vi "RestoreUISettings.vi"(8 "Error In":errorcluster, 11 "UI References":T1) -> (0 "Error Out":errorcluster)   [LabVIEW 2017, in "Client.lvlib" / "UI_API.lvlib"]
uses:
  UI_API.lvlib
  NI_LVConfig.lvlib
  Client.lvlib
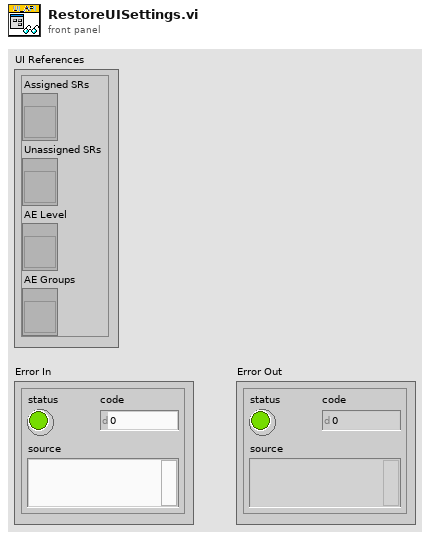
[diagram p1: front panel]
types:
  T1 = cluster{"Assigned SRs":refnum<vi>, "Unassigned SRs":refnum<vi>, "AE Level":refnum<vi>, "AE Groups":refnum<vi>}
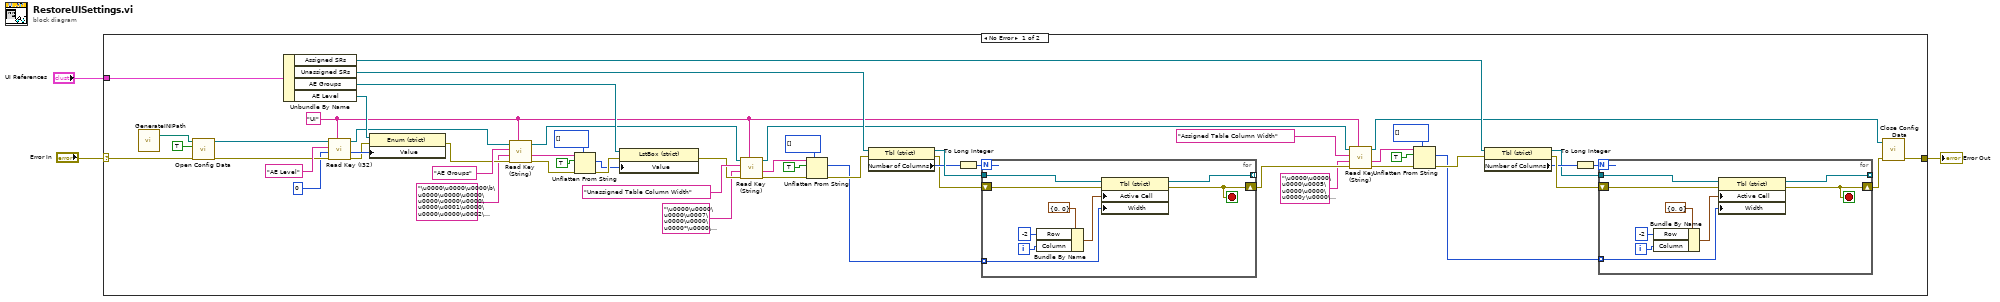
[diagram p0: block diagram]
diagram:
  n1 = case shown="No Error" "Error In" {
    selector: "Error In" -> [w58 w78]
    tunnel: "UI References" -> [w57 _]
    tunnel: [w54 w78] -> w1
    frame No Error {
      w24 = "UI" ("section")
      n2 = call "GenerateINIPath.vi"() -> ("INI Path"=w4:path)  [unwired: 11 in]
      n3 = call "Open Config Data.vi"("error in (no error)"=w58, "create file if necessary (T)"=TRUE ("create file if necessary? (T)"), "configuration file path"=w4) -> ("error out"=w45:errorcluster, "refnum"=w48:refnum<k1>)  [unwired: 6 in, 1 out]
      n4 = Unbundle By Name(w57) -> ("Assigned SRs"=w12:refnum<vi>, "Unassigned SRs"=w53:refnum<vi>, "AE Groups"=w55:refnum<vi>, "AE Level"=w56:refnum<vi>)
      n5 = call "Read Key (I32).vi"("section"=w24, "error in (no error)"=w45, "default value"=0, "key"="AE Level", "refnum"=w48) -> ("error out"=w44:errorcluster, "value"=w46:i32, "refnum out"=w40:refnum<k1>)  [unwired: 3 in, 1 out]
      n6 = property class="Enum (strict)"(reference=w56, error in=w44, "Value"=w46) -> (error out=w41:errorcluster)  [unwired: 1 out]
      n7 = call "Read Key (String).vi"("section"=w24, "error in (no error)"=w41, "default value"="\u0000\u0000\u0000\b\u0000\u0000\u0000\u0000\u0000\u0000\u0000\u0001\u0000\u0000\u0000\u0002\u0000\u0000\u0000\u0003\u0000\u0000\u0000\u0004\u0000\u0000\u0000\u0005\u0000\u0000\u0000\u0006\u0000\u0000\u0000\u0007", "key"="AE Groups", "refnum"=w40) -> ("error out"=w37:errorcluster, "value"=w38:string, "refnum out"=w32:refnum<k1>)  [unwired: 3 in, 1 out]
      n8 = Unflatten From String(type=i32[] [] ("Value"), binary string=w38, data includes array or string size? (T)=TRUE, error in (no error)=w37) -> (value=w35:i32[], error out=w36:errorcluster)  [unwired: 1 in, 1 out]
      n9 = property class="LstBox (strict)"(reference=w55, error in=w36, "Value"=w35) -> (error out=w33:errorcluster)  [unwired: 1 out]
      n10 = call "Read Key (String).vi"("section"=w24, "error in (no error)"=w33, "default value"="\u0000\u0000\u0000\u0007\u0000\u0000\u0000*\u0000\u0000\u0000F\u0000\u0000\u0000L\u0000\u0000\u0001\u0000\u0000\u0001\u0013\u0000\u0000\u0000E\u0000\u0000\u0000Z", "key"="Unassigned Table Column Width", "refnum"=w32) -> ("error out"=w28:errorcluster, "value"=w29:string, "refnum out"=w22:refnum<k1>)  [unwired: 3 in, 1 out]
      n11 = Unflatten From String(type=u32[] [], binary string=w29, data includes array or string size? (T)=TRUE, error in (no error)=w28) -> (value=w26:u32[], error out=w27:errorcluster)  [unwired: 1 in, 1 out]
      n12 = property class="Tbl (strict)"(reference=w53, error in=w27) -> (reference out=w52:refnum<vi>, error out=w49:errorcluster, "Number of Columns"=w51:u32)
      n13 = To Long Integer(number=w51) -> (32bit integer=w50:i32)
      n14 = for {
        N: w50 -> [_]
        shift-right: [w71] -> w25
        shift-left: w49 -> [w72]
        tunnel: w52 -> [w77]
        tunnel: [w73] -> _ mode=indexing
        tunnel: w26 -> [w70] mode=indexing
        i -> [w69]
        stop <- w71 stop-if-true
        n15 = Bundle By Name(cluster=cluster{"Row":i32, "Column":i32} {"Row"=0, "Column"=0} ("Active Cell:Active Cell"), "Row"=-2, "Column"=w69) -> (w74:cluster{"Row":i32, "Column":i32})
        n16 = property class="Tbl (strict)"(reference=w77, error in=w72, "Active Cell"=w74, "Width"=w70) -> (reference out=w73:refnum<vi>, error out=w71:errorcluster)
      }
      n17 = call "Read Key (String).vi"("section"=w24, "error in (no error)"=w25, "default value"="\u0000\u0000\u0000\u0005\u0000\u0000\u0000y\u0000\u0000\u0000;\u0000\u0000\u0001n\u0000\u0000\u0001\u0000\u0000\u0001\u0013", "key"="Assigned Table Column Width", "refnum"=w22) -> ("error out"=w15:errorcluster, "value"=w14:string, "refnum out"=w9:refnum<k1>)  [unwired: 3 in, 1 out]
      n18 = Unflatten From String(type=u32[] [], binary string=w14, data includes array or string size? (T)=TRUE, error in (no error)=w15) -> (value=w11:u32[], error out=w13:errorcluster)  [unwired: 1 in, 1 out]
      n19 = property class="Tbl (strict)"(reference=w12, error in=w13) -> (reference out=w18:refnum<vi>, error out=w21:errorcluster, "Number of Columns"=w19:u32)
      n20 = To Long Integer(number=w19) -> (32bit integer=w20:i32)
      n21 = for {
        N: w20 -> [_]
        shift-right: [w62] -> w10
        shift-left: w21 -> [w63]
        tunnel: w18 -> [w68]
        tunnel: [w64] -> _ mode=indexing
        tunnel: w11 -> [w60] mode=indexing
        i -> [w61]
        stop <- w62 stop-if-true
        n22 = Bundle By Name(cluster=cluster{"Row":i32, "Column":i32} {"Row"=0, "Column"=0} ("Active Cell:Active Cell"), "Row"=-2, "Column"=w61) -> (w65:cluster{"Row":i32, "Column":i32})
        n23 = property class="Tbl (strict)"(reference=w68, error in=w63, "Active Cell"=w65, "Width"=w60) -> (reference out=w64:refnum<vi>, error out=w62:errorcluster)
      }
      n24 = call "Close Config Data.vi"("error in (no error)"=w10, "refnum"=w9) -> ("error out"=w54:errorcluster)  [unwired: 8 in, 1 out]
    }
    frame Error {
    }
  }
  "Error Out" <- w1
